vi "A1_图像处理结果.vi"(0 "Image In":T3(plugin-control), 5 "ParamsUI":T1={"IsNorImage"=FALSE, "Exposure Values"=0, "ImagePath"=path "", " Step1 Range"={"Lower value"=117.0, "Upper value"=255.0}, "Step2 Selection Values"=[{"Measurement Parameter"=5, "Range Lower Value"=223.0, "Range Upper Value"=707.0, "Range"=FALSE, "Measurement Type"=FALSE}, {"Measurement Parameter"=4, "Range Lower Value"=0.0, "Range Upper Value"=0.0, "Range"=FALSE, "Measurement Type"=FALSE}], "Step2 Keep/Remove Particles"=TRUE, "Step3 Selection Values 2"=[{"Measurement Parameter"=35, "Range Lower Value"=700.0, "Range Upper Value"=16882.0, "Range"=FALSE, "Measurement Type"=FALSE}], "Step3Keep/Remove Particles 2"=TRUE, "Step4 Selection Values"=[{"Measurement Parameter"=35, "Range Lower Value"=0.0, "Range Upper Value"=393.0, "Range"=FALSE, "Measurement Type"=FALSE}], "Step4 Keep/Remove Particles"=TRUE, "Step5Selection Values"=[{"Measurement Parameter"=2, "Range Lower Value"=564.0, "Range Upper Value"=2005.0, "Range"=FALSE, "Measurement Type"=FALSE}], "Step5 Keep/Remove Particles"=TRUE, "Inspection Number"=0} caption="参数界面" {"Step5Selection Values"."Measurement Parameter" items=["Center of Mass X", "Center of Mass Y", "First Pixel X", "First Pixel Y", "Bounding Rect Left", "Bounding Rect Top", "Bounding Rect Right", "Bounding Rect Bottom", "Max Feret Diameter Start X", "Max Feret Diameter Start Y", "Max Feret Diameter End X", "Max Feret Diameter End Y", "Max Horiz. Segment Length Left", "Max Horiz. Segment Length Right", "Max Horiz. Segment Length Row", "-", "Bounding Rect Width", "Bounding Rect Height", "Bounding Rect Diagonal", "Perimeter", "Convex Hull Perimeter", "Holes' Perimeter", "Max Feret Diameter", "Equivalent Ellipse Major Axis", "Equivalent Ellipse Minor Axis", "Equivalent Ellipse Minor Axis (Feret)", "Equivalent Rect Long Side", "Equivalent Rect Short Side", "Equivalent Rect Diagonal", "Equivalent Rect Short Side (Feret)", "Average Horiz. Segment Length", "Average Vert. Segment Length", "Hydraulic Radius", "Waddel Disk Diameter", "-", "Area", "Holes' Area", "Particle & Holes' Area", "Convex Hull Area", "Image Area", "-", "Number of Holes", "Number of Horiz. Segments", "Number of Vert. Segments", "-", "Orientation", "Max Feret Diameter Orientation", "-", "% Area/Image Area", "% Area/(Particle & Holes' Area)", "Ratio of Equivalent Ellipse Axes", "Ratio of Equivalent Rect Sides", "-", "Elongation Factor", "Compactness Factor", "Heywood Circularity Factor", "Type Factor", "-", "Sum X", "Sum Y", "Sum XX", "Sum XY", "Sum YY", "Sum XXX", "Sum XXY", "Sum XYY", "Sum YYY", "-", "Moment of Inertia XX", "Moment of Inertia XY", "Moment of Inertia YY", "Moment of Inertia XXX", "Moment of Inertia XXY", "Moment of Inertia XYY", "Moment of Inertia YYY", "Norm. Moment of Inertia XX", "Norm. Moment of Inertia XY", "Norm. Moment of Inertia YY", "Norm. Moment of Inertia XXX", "Norm. Moment of Inertia XXY", "Norm. Moment of Inertia XYY", "Norm. Moment of Inertia YYY", "Hu Moment 1", "Hu Moment 2", "Hu Moment 3", "Hu Moment 4", "Hu Moment 5", "Hu Moment 6", "Hu Moment 7"]; "Step4 Selection Values"."Measurement Parameter" items=["Center of Mass X", "Center of Mass Y", "First Pixel X", "First Pixel Y", "Bounding Rect Left", "Bounding Rect Top", "Bounding Rect Right", "Bounding Rect Bottom", "Max Feret Diameter Start X", "Max Feret Diameter Start Y", "Max Feret Diameter End X", "Max Feret Diameter End Y", "Max Horiz. Segment Length Left", "Max Horiz. Segment Length Right", "Max Horiz. Segment Length Row", "-", "Bounding Rect Width", "Bounding Rect Height", "Bounding Rect Diagonal", "Perimeter", "Convex Hull Perimeter", "Holes' Perimeter", "Max Feret Diameter", "Equivalent Ellipse Major Axis", "Equivalent Ellipse Minor Axis", "Equivalent Ellipse Minor Axis (Feret)", "Equivalent Rect Long Side", "Equivalent Rect Short Side", "Equivalent Rect Diagonal", "Equivalent Rect Short Side (Feret)", "Average Horiz. Segment Length", "Average Vert. Segment Length", "Hydraulic Radius", "Waddel Disk Diameter", "-", "Area", "Holes' Area", "Particle & Holes' Area", "Convex Hull Area", "Image Area", "-", "Number of Holes", "Number of Horiz. Segments", "Number of Vert. Segments", "-", "Orientation", "Max Feret Diameter Orientation", "-", "% Area/Image Area", "% Area/(Particle & Holes' Area)", "Ratio of Equivalent Ellipse Axes", "Ratio of Equivalent Rect Sides", "-", "Elongation Factor", "Compactness Factor", "Heywood Circularity Factor", "Type Factor", "-", "Sum X", "Sum Y", "Sum XX", "Sum XY", "Sum YY", "Sum XXX", "Sum XXY", "Sum XYY", "Sum YYY", "-", "Moment of Inertia XX", "Moment of Inertia XY", "Moment of Inertia YY", "Moment of Inertia XXX", "Moment of Inertia XXY", "Moment of Inertia XYY", "Moment of Inertia YYY", "Norm. Moment of Inertia XX", "Norm. Moment of Inertia XY", "Norm. Moment of Inertia YY", "Norm. Moment of Inertia XXX", "Norm. Moment of Inertia XXY", "Norm. Moment of Inertia XYY", "Norm. Moment of Inertia YYY", "Hu Moment 1", "Hu Moment 2", "Hu Moment 3", "Hu Moment 4", "Hu Moment 5", "Hu Moment 6", "Hu Moment 7"]; "Step3 Selection Values 2"."Measurement Parameter" items=["Center of Mass X", "Center of Mass Y", "First Pixel X", "First Pixel Y", "Bounding Rect Left", "Bounding Rect Top", "Bounding Rect Right", "Bounding Rect Bottom", "Max Feret Diameter Start X", "Max Feret Diameter Start Y", "Max Feret Diameter End X", "Max Feret Diameter End Y", "Max Horiz. Segment Length Left", "Max Horiz. Segment Length Right", "Max Horiz. Segment Length Row", "-", "Bounding Rect Width", "Bounding Rect Height", "Bounding Rect Diagonal", "Perimeter", "Convex Hull Perimeter", "Holes' Perimeter", "Max Feret Diameter", "Equivalent Ellipse Major Axis", "Equivalent Ellipse Minor Axis", "Equivalent Ellipse Minor Axis (Feret)", "Equivalent Rect Long Side", "Equivalent Rect Short Side", "Equivalent Rect Diagonal", "Equivalent Rect Short Side (Feret)", "Average Horiz. Segment Length", "Average Vert. Segment Length", "Hydraulic Radius", "Waddel Disk Diameter", "-", "Area", "Holes' Area", "Particle & Holes' Area", "Convex Hull Area", "Image Area", "-", "Number of Holes", "Number of Horiz. Segments", "Number of Vert. Segments", "-", "Orientation", "Max Feret Diameter Orientation", "-", "% Area/Image Area", "% Area/(Particle & Holes' Area)", "Ratio of Equivalent Ellipse Axes", "Ratio of Equivalent Rect Sides", "-", "Elongation Factor", "Compactness Factor", "Heywood Circularity Factor", "Type Factor", "-", "Sum X", "Sum Y", "Sum XX", "Sum XY", "Sum YY", "Sum XXX", "Sum XXY", "Sum XYY", "Sum YYY", "-", "Moment of Inertia XX", "Moment of Inertia XY", "Moment of Inertia YY", "Moment of Inertia XXX", "Moment of Inertia XXY", "Moment of Inertia XYY", "Moment of Inertia YYY", "Norm. Moment of Inertia XX", "Norm. Moment of Inertia XY", "Norm. Moment of Inertia YY", "Norm. Moment of Inertia XXX", "Norm. Moment of Inertia XXY", "Norm. Moment of Inertia XYY", "Norm. Moment of Inertia YYY", "Hu Moment 1", "Hu Moment 2", "Hu Moment 3", "Hu Moment 4", "Hu Moment 5", "Hu Moment 6", "Hu Moment 7"]; "Step2 Selection Values"."Measurement Parameter" items=["Center of Mass X", "Center of Mass Y", "First Pixel X", "First Pixel Y", "Bounding Rect Left", "Bounding Rect Top", "Bounding Rect Right", "Bounding Rect Bottom", "Max Feret Diameter Start X", "Max Feret Diameter Start Y", "Max Feret Diameter End X", "Max Feret Diameter End Y", "Max Horiz. Segment Length Left", "Max Horiz. Segment Length Right", "Max Horiz. Segment Length Row", "-", "Bounding Rect Width", "Bounding Rect Height", "Bounding Rect Diagonal", "Perimeter", "Convex Hull Perimeter", "Holes' Perimeter", "Max Feret Diameter", "Equivalent Ellipse Major Axis", "Equivalent Ellipse Minor Axis", "Equivalent Ellipse Minor Axis (Feret)", "Equivalent Rect Long Side", "Equivalent Rect Short Side", "Equivalent Rect Diagonal", "Equivalent Rect Short Side (Feret)", "Average Horiz. Segment Length", "Average Vert. Segment Length", "Hydraulic Radius", "Waddel Disk Diameter", "-", "Area", "Holes' Area", "Particle & Holes' Area", "Convex Hull Area", "Image Area", "-", "Number of Holes", "Number of Horiz. Segments", "Number of Vert. Segments", "-", "Orientation", "Max Feret Diameter Orientation", "-", "% Area/Image Area", "% Area/(Particle & Holes' Area)", "Ratio of Equivalent Ellipse Axes", "Ratio of Equivalent Rect Sides", "-", "Elongation Factor", "Compactness Factor", "Heywood Circularity Factor", "Type Factor", "-", "Sum X", "Sum Y", "Sum XX", "Sum XY", "Sum YY", "Sum XXX", "Sum XXY", "Sum XYY", "Sum YYY", "-", "Moment of Inertia XX", "Moment of Inertia XY", "Moment of Inertia YY", "Moment of Inertia XXX", "Moment of Inertia XXY", "Moment of Inertia XYY", "Moment of Inertia YYY", "Norm. Moment of Inertia XX", "Norm. Moment of Inertia XY", "Norm. Moment of Inertia YY", "Norm. Moment of Inertia XXX", "Norm. Moment of Inertia XXY", "Norm. Moment of Inertia XYY", "Norm. Moment of Inertia YYY", "Hu Moment 1", "Hu Moment 2", "Hu Moment 3", "Hu Moment 4", "Hu Moment 5", "Hu Moment 6", "Hu Moment 7"]; "Exposure Values" scale=0.0..200000.0}, 11 "error in":errorcluster) -> (4 "Image Out":T3(plugin-control), 6 "Particle Measurements (Real-World)":dbl[][](array[numeric]) format="%.2f", 15 "error out":errorcluster)   [LabVIEW 2015]
uses:
  <vilib>/vision/NI_Vision_Development_Module.lvlib
panel:
  in  "Step5 Keep/Remove Particles":bool=TRUE
  in  "Step5Selection Values":T2(array[cluster])=[{"Measurement Parameter"=2, "Range Lower Value"=564.0, "Range Upper Value"=2005.0, "Range"=FALSE, "Measurement Type"=FALSE}] {"Measurement Parameter" items=["Center of Mass X", "Center of Mass Y", "First Pixel X", "First Pixel Y", "Bounding Rect Left", "Bounding Rect Top", "Bounding Rect Right", "Bounding Rect Bottom", "Max Feret Diameter Start X", "Max Feret Diameter Start Y", "Max Feret Diameter End X", "Max Feret Diameter End Y", "Max Horiz. Segment Length Left", "Max Horiz. Segment Length Right", "Max Horiz. Segment Length Row", "-", "Bounding Rect Width", "Bounding Rect Height", "Bounding Rect Diagonal", "Perimeter", "Convex Hull Perimeter", "Holes' Perimeter", "Max Feret Diameter", "Equivalent Ellipse Major Axis", "Equivalent Ellipse Minor Axis", "Equivalent Ellipse Minor Axis (Feret)", "Equivalent Rect Long Side", "Equivalent Rect Short Side", "Equivalent Rect Diagonal", "Equivalent Rect Short Side (Feret)", "Average Horiz. Segment Length", "Average Vert. Segment Length", "Hydraulic Radius", "Waddel Disk Diameter", "-", "Area", "Holes' Area", "Particle & Holes' Area", "Convex Hull Area", "Image Area", "-", "Number of Holes", "Number of Horiz. Segments", "Number of Vert. Segments", "-", "Orientation", "Max Feret Diameter Orientation", "-", "% Area/Image Area", "% Area/(Particle & Holes' Area)", "Ratio of Equivalent Ellipse Axes", "Ratio of Equivalent Rect Sides", "-", "Elongation Factor", "Compactness Factor", "Heywood Circularity Factor", "Type Factor", "-", "Sum X", "Sum Y", "Sum XX", "Sum XY", "Sum YY", "Sum XXX", "Sum XXY", "Sum XYY", "Sum YYY", "-", "Moment of Inertia XX", "Moment of Inertia XY", "Moment of Inertia YY", "Moment of Inertia XXX", "Moment of Inertia XXY", "Moment of Inertia XYY", "Moment of Inertia YYY", "Norm. Moment of Inertia XX", "Norm. Moment of Inertia XY", "Norm. Moment of Inertia YY", "Norm. Moment of Inertia XXX", "Norm. Moment of Inertia XXY", "Norm. Moment of Inertia XYY", "Norm. Moment of Inertia YYY", "Hu Moment 1", "Hu Moment 2", "Hu Moment 3", "Hu Moment 4", "Hu Moment 5", "Hu Moment 6", "Hu Moment 7"]}
  in  "Step4Keep/Remove Particles":bool=TRUE
  in  "Step4 Selection Values":T2(array[cluster])=[{"Measurement Parameter"=35, "Range Lower Value"=0.0, "Range Upper Value"=393.0, "Range"=FALSE, "Measurement Type"=FALSE}] {"Measurement Parameter" items=["Center of Mass X", "Center of Mass Y", "First Pixel X", "First Pixel Y", "Bounding Rect Left", "Bounding Rect Top", "Bounding Rect Right", "Bounding Rect Bottom", "Max Feret Diameter Start X", "Max Feret Diameter Start Y", "Max Feret Diameter End X", "Max Feret Diameter End Y", "Max Horiz. Segment Length Left", "Max Horiz. Segment Length Right", "Max Horiz. Segment Length Row", "-", "Bounding Rect Width", "Bounding Rect Height", "Bounding Rect Diagonal", "Perimeter", "Convex Hull Perimeter", "Holes' Perimeter", "Max Feret Diameter", "Equivalent Ellipse Major Axis", "Equivalent Ellipse Minor Axis", "Equivalent Ellipse Minor Axis (Feret)", "Equivalent Rect Long Side", "Equivalent Rect Short Side", "Equivalent Rect Diagonal", "Equivalent Rect Short Side (Feret)", "Average Horiz. Segment Length", "Average Vert. Segment Length", "Hydraulic Radius", "Waddel Disk Diameter", "-", "Area", "Holes' Area", "Particle & Holes' Area", "Convex Hull Area", "Image Area", "-", "Number of Holes", "Number of Horiz. Segments", "Number of Vert. Segments", "-", "Orientation", "Max Feret Diameter Orientation", "-", "% Area/Image Area", "% Area/(Particle & Holes' Area)", "Ratio of Equivalent Ellipse Axes", "Ratio of Equivalent Rect Sides", "-", "Elongation Factor", "Compactness Factor", "Heywood Circularity Factor", "Type Factor", "-", "Sum X", "Sum Y", "Sum XX", "Sum XY", "Sum YY", "Sum XXX", "Sum XXY", "Sum XYY", "Sum YYY", "-", "Moment of Inertia XX", "Moment of Inertia XY", "Moment of Inertia YY", "Moment of Inertia XXX", "Moment of Inertia XXY", "Moment of Inertia XYY", "Moment of Inertia YYY", "Norm. Moment of Inertia XX", "Norm. Moment of Inertia XY", "Norm. Moment of Inertia YY", "Norm. Moment of Inertia XXX", "Norm. Moment of Inertia XXY", "Norm. Moment of Inertia XYY", "Norm. Moment of Inertia YYY", "Hu Moment 1", "Hu Moment 2", "Hu Moment 3", "Hu Moment 4", "Hu Moment 5", "Hu Moment 6", "Hu Moment 7"]}
  in  "Step3Keep/Remove Particles 2":bool=TRUE
  in  "Step3 Selection Values 2":T2(array[cluster])=[{"Measurement Parameter"=35, "Range Lower Value"=700.0, "Range Upper Value"=16882.0, "Range"=FALSE, "Measurement Type"=FALSE}] {"Measurement Parameter" items=["Center of Mass X", "Center of Mass Y", "First Pixel X", "First Pixel Y", "Bounding Rect Left", "Bounding Rect Top", "Bounding Rect Right", "Bounding Rect Bottom", "Max Feret Diameter Start X", "Max Feret Diameter Start Y", "Max Feret Diameter End X", "Max Feret Diameter End Y", "Max Horiz. Segment Length Left", "Max Horiz. Segment Length Right", "Max Horiz. Segment Length Row", "-", "Bounding Rect Width", "Bounding Rect Height", "Bounding Rect Diagonal", "Perimeter", "Convex Hull Perimeter", "Holes' Perimeter", "Max Feret Diameter", "Equivalent Ellipse Major Axis", "Equivalent Ellipse Minor Axis", "Equivalent Ellipse Minor Axis (Feret)", "Equivalent Rect Long Side", "Equivalent Rect Short Side", "Equivalent Rect Diagonal", "Equivalent Rect Short Side (Feret)", "Average Horiz. Segment Length", "Average Vert. Segment Length", "Hydraulic Radius", "Waddel Disk Diameter", "-", "Area", "Holes' Area", "Particle & Holes' Area", "Convex Hull Area", "Image Area", "-", "Number of Holes", "Number of Horiz. Segments", "Number of Vert. Segments", "-", "Orientation", "Max Feret Diameter Orientation", "-", "% Area/Image Area", "% Area/(Particle & Holes' Area)", "Ratio of Equivalent Ellipse Axes", "Ratio of Equivalent Rect Sides", "-", "Elongation Factor", "Compactness Factor", "Heywood Circularity Factor", "Type Factor", "-", "Sum X", "Sum Y", "Sum XX", "Sum XY", "Sum YY", "Sum XXX", "Sum XXY", "Sum XYY", "Sum YYY", "-", "Moment of Inertia XX", "Moment of Inertia XY", "Moment of Inertia YY", "Moment of Inertia XXX", "Moment of Inertia XXY", "Moment of Inertia XYY", "Moment of Inertia YYY", "Norm. Moment of Inertia XX", "Norm. Moment of Inertia XY", "Norm. Moment of Inertia YY", "Norm. Moment of Inertia XXX", "Norm. Moment of Inertia XXY", "Norm. Moment of Inertia XYY", "Norm. Moment of Inertia YYY", "Hu Moment 1", "Hu Moment 2", "Hu Moment 3", "Hu Moment 4", "Hu Moment 5", "Hu Moment 6", "Hu Moment 7"]}
  in  "Step2 Keep/Remove Particles":bool=TRUE
  in  "Step2 Selection Values":T2(array[cluster])=[{"Measurement Parameter"=5, "Range Lower Value"=223.0, "Range Upper Value"=707.0, "Range"=FALSE, "Measurement Type"=FALSE}, {"Measurement Parameter"=4, "Range Lower Value"=0.0, "Range Upper Value"=0.0, "Range"=FALSE, "Measurement Type"=FALSE}] {"Measurement Parameter" items=["Center of Mass X", "Center of Mass Y", "First Pixel X", "First Pixel Y", "Bounding Rect Left", "Bounding Rect Top", "Bounding Rect Right", "Bounding Rect Bottom", "Max Feret Diameter Start X", "Max Feret Diameter Start Y", "Max Feret Diameter End X", "Max Feret Diameter End Y", "Max Horiz. Segment Length Left", "Max Horiz. Segment Length Right", "Max Horiz. Segment Length Row", "-", "Bounding Rect Width", "Bounding Rect Height", "Bounding Rect Diagonal", "Perimeter", "Convex Hull Perimeter", "Holes' Perimeter", "Max Feret Diameter", "Equivalent Ellipse Major Axis", "Equivalent Ellipse Minor Axis", "Equivalent Ellipse Minor Axis (Feret)", "Equivalent Rect Long Side", "Equivalent Rect Short Side", "Equivalent Rect Diagonal", "Equivalent Rect Short Side (Feret)", "Average Horiz. Segment Length", "Average Vert. Segment Length", "Hydraulic Radius", "Waddel Disk Diameter", "-", "Area", "Holes' Area", "Particle & Holes' Area", "Convex Hull Area", "Image Area", "-", "Number of Holes", "Number of Horiz. Segments", "Number of Vert. Segments", "-", "Orientation", "Max Feret Diameter Orientation", "-", "% Area/Image Area", "% Area/(Particle & Holes' Area)", "Ratio of Equivalent Ellipse Axes", "Ratio of Equivalent Rect Sides", "-", "Elongation Factor", "Compactness Factor", "Heywood Circularity Factor", "Type Factor", "-", "Sum X", "Sum Y", "Sum XX", "Sum XY", "Sum YY", "Sum XXX", "Sum XXY", "Sum XYY", "Sum YYY", "-", "Moment of Inertia XX", "Moment of Inertia XY", "Moment of Inertia YY", "Moment of Inertia XXX", "Moment of Inertia XXY", "Moment of Inertia XYY", "Moment of Inertia YYY", "Norm. Moment of Inertia XX", "Norm. Moment of Inertia XY", "Norm. Moment of Inertia YY", "Norm. Moment of Inertia XXX", "Norm. Moment of Inertia XXY", "Norm. Moment of Inertia XYY", "Norm. Moment of Inertia YYY", "Hu Moment 1", "Hu Moment 2", "Hu Moment 3", "Hu Moment 4", "Hu Moment 5", "Hu Moment 6", "Hu Moment 7"]}
  in  "Step1 Range In":cluster{"Lower value":sgl, "Upper value":sgl}={"Lower value"=117.0, "Upper value"=255.0}
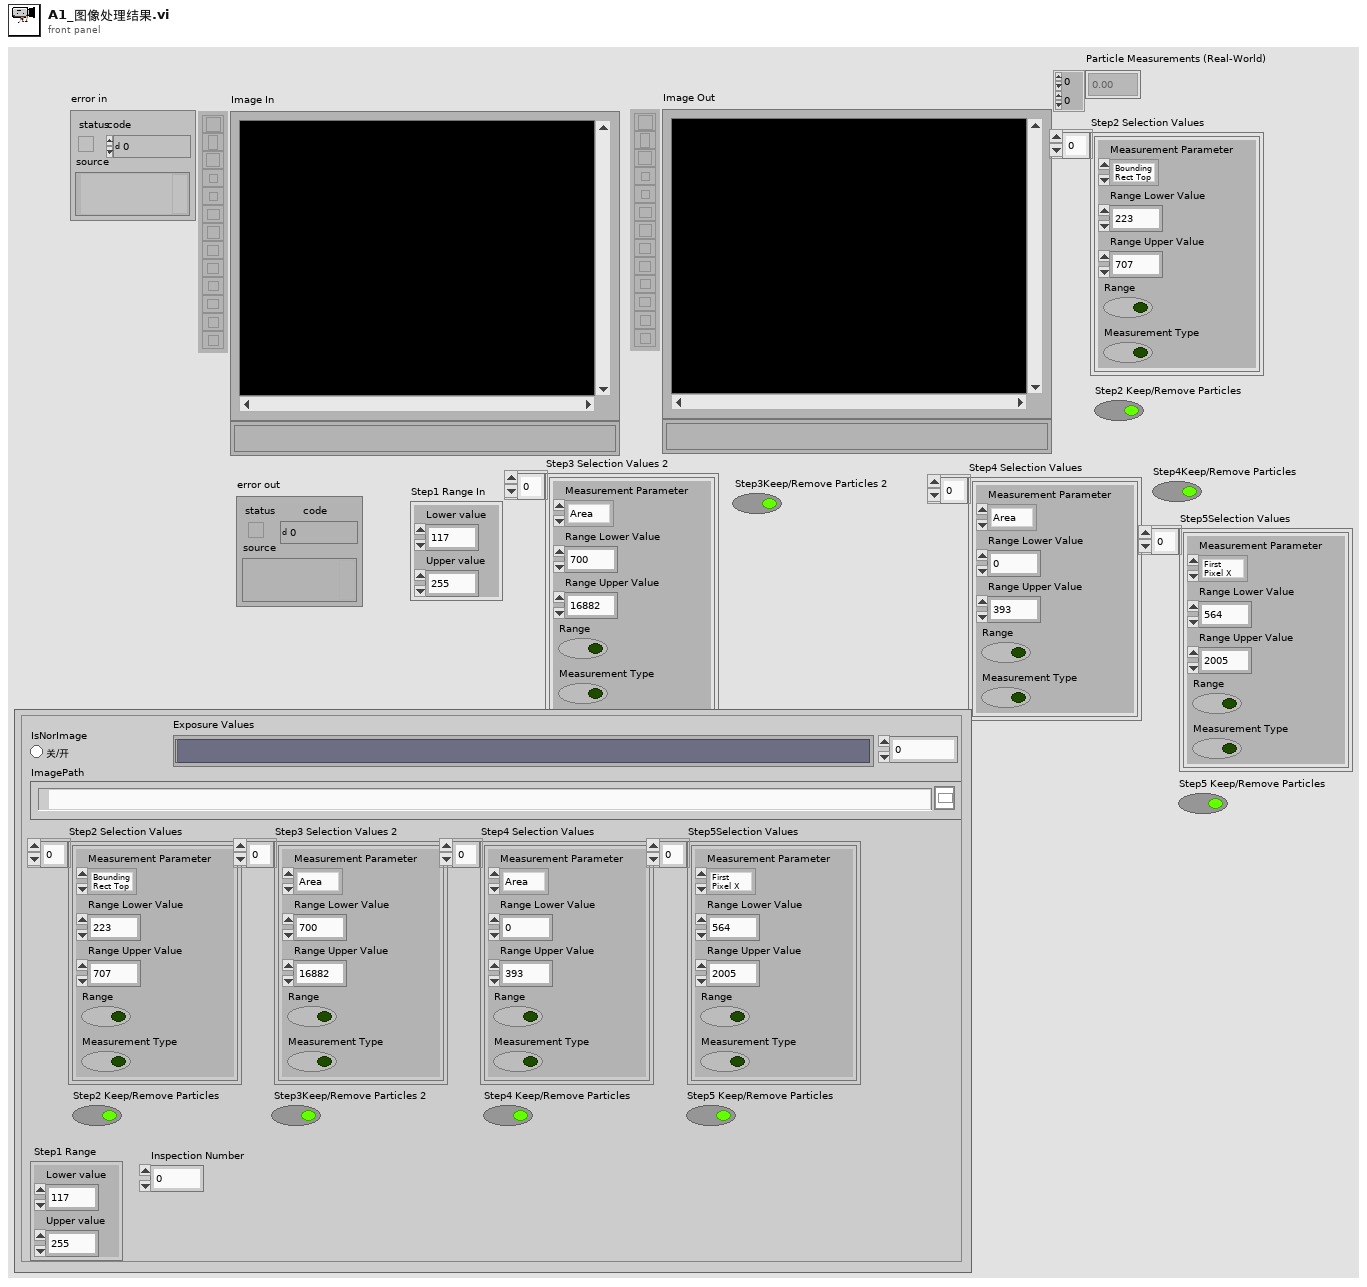
[diagram p1: front panel]
types:
  T1 = cluster{"IsNorImage":bool, "Exposure Values":u32, "ImagePath":path, " Step1 Range":cluster{"Lower value":sgl, "Upper value":sgl}, "Step2 Selection Values":cluster{"Measurement Parameter":i32, "Range Lower Value":dbl, "Range Upper Value":dbl, "Range":bool, "Measurement Type":bool}[], "Step2 Keep/Remove Particles":bool, "Step3 Selection Values 2":cluster{"Measurement Parameter":i32, "Range Lower Value":dbl, "Range Upper Value":dbl, "Range":bool, "Measurement Type":bool}[], "Step3Keep/Remove Particles 2":bool, "Step4 Selection Values":cluster{"Measurement Parameter":i32, "Range Lower Value":dbl, "Range Upper Value":dbl, "Range":bool, "Measurement Type":bool}[], "Step4 Keep/Remove Particles":bool, "Step5Selection Values":cluster{"Measurement Parameter":i32, "Range Lower Value":dbl, "Range Upper Value":dbl, "Range":bool, "Measurement Type":bool}[], "Step5 Keep/Remove Particles":bool, "Inspection Number":i32}
  T2 = cluster{"Measurement Parameter":i32, "Range Lower Value":dbl, "Range Upper Value":dbl, "Range":bool, "Measurement Type":bool}[]
  T3 = typedef "IMAQ Image.ctl" = refnum<image>
  T4 = enum32{"Differentiation", "Gradient", "Prewitt", "Roberts", "Sigma", "Sobel"}
  T5 = enum32{"AutoM", "Close", "Dilate", "Erode", "Gradient", "Gradient in", "Gradient out", "HitMiss", "Open", "PClose", "POpen", "Thick", "Thin"}
  T6 = cluster{"histogram":u32[], "Minimal Value":sgl, "Maximal Value":sgl, "Starting Value":sgl, "Interval Width":sgl, "Mean Value":sgl, "Standard  Variation":sgl, "Area (pixels)":i32}
  T7 = typedef "Image Type" = u32
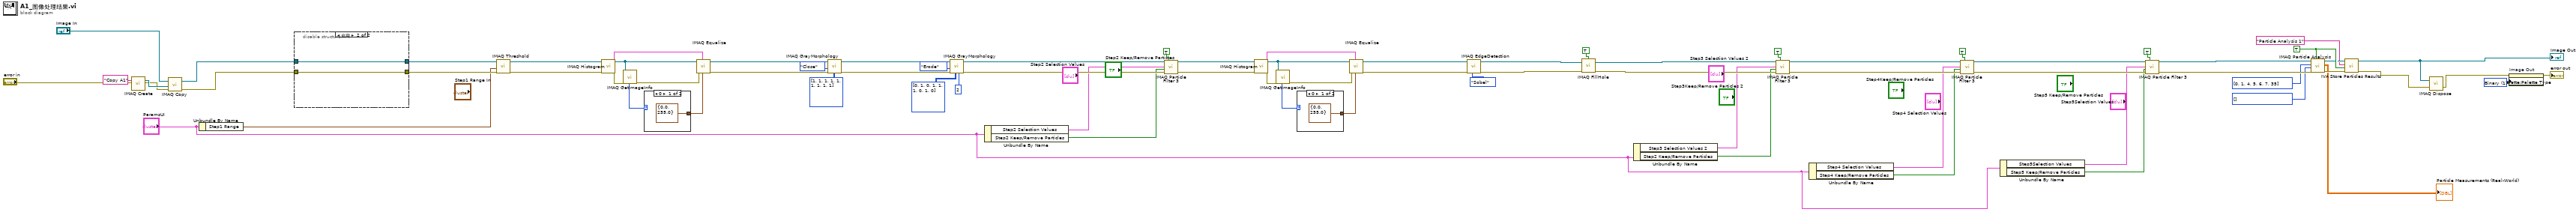
[diagram p0: block diagram]
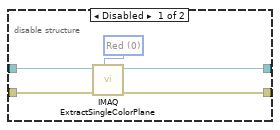
[diagram p2: hidden frame]
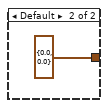
[diagram p3: hidden frame]
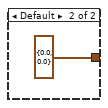
[diagram p4: hidden frame]
diagram:
  w21 = u32 1 items=["Grayscale", "Binary", "Gradient", "Rainbow", "Temperature", "User Defined", "Binary 16 Bit", "Gradient 16 Bit", "Rainbow 16 Bit", "Temperature 16 Bit", "User Defined 16 Bit"] ("Palette Type")
  w28 = i32[] [] items=["Center of Mass X", "Center of Mass Y", "First Pixel X", "First Pixel Y", "Bounding Rect Left", "Bounding Rect Top", "Bounding Rect Right", "Bounding Rect Bottom", "Max Feret Diameter Start X", "Max Feret Diameter Start Y", "Max Feret Diameter End X", "Max Feret Diameter End Y", "Max Horiz. Segment Length Left", "Max Horiz. Segment Length Right", "Max Horiz. Segment Length Row", "-", "Bounding Rect Width", "Bounding Rect Height", "Bounding Rect Diagonal", "Perimeter", "Convex Hull Perimeter", "Holes' Perimeter", "Max Feret Diameter", "Equivalent Ellipse Major Axis", "Equivalent Ellipse Minor Axis", "Equivalent Ellipse Minor Axis (Feret)", "Equivalent Rect Long Side", "Equivalent Rect Short Side", "Equivalent Rect Diagonal", "Equivalent Rect Short Side (Feret)", "Average Horiz. Segment Length", "Average Vert. Segment Length", "Hydraulic Radius", "Waddel Disk Diameter", "-", "Area", "Holes' Area", "Particle & Holes' Area", "Convex Hull Area", "Image Area", "-", "Number of Holes", "Number of Horiz. Segments", "Number of Vert. Segments", "-", "Orientation", "Max Feret Diameter Orientation", "-", "% Area/Image Area", "% Area/(Particle & Holes' Area)", "Ratio of Equivalent Ellipse Axes", "Ratio of Equivalent Rect Sides", "-", "Elongation Factor", "Compactness Factor", "Heywood Circularity Factor", "Type Factor", "-", "Sum X", "Sum Y", "Sum XX", "Sum XY", "Sum YY", "Sum XXX", "Sum XXY", "Sum XYY", "Sum YYY", "-", "Moment of Inertia XX", "Moment of Inertia XY", "Moment of Inertia YY", "Moment of Inertia XXX", "Moment of Inertia XXY", "Moment of Inertia XYY", "Moment of Inertia YYY", "Norm. Moment of Inertia XX", "Norm. Moment of Inertia XY", "Norm. Moment of Inertia YY", "Norm. Moment of Inertia XXX", "Norm. Moment of Inertia XXY", "Norm. Moment of Inertia XYY", "Norm. Moment of Inertia YYY", "Hu Moment 1", "Hu Moment 2", "Hu Moment 3", "Hu Moment 4", "Hu Moment 5", "Hu Moment 6", "Hu Moment 7"] ("Real-World Measurements")
  w29 = i32[] [0, 1, 4, 5, 6, 7, 35] items=["Center of Mass X", "Center of Mass Y", "First Pixel X", "First Pixel Y", "Bounding Rect Left", "Bounding Rect Top", "Bounding Rect Right", "Bounding Rect Bottom", "Max Feret Diameter Start X", "Max Feret Diameter Start Y", "Max Feret Diameter End X", "Max Feret Diameter End Y", "Max Horiz. Segment Length Left", "Max Horiz. Segment Length Right", "Max Horiz. Segment Length Row", "-", "Bounding Rect Width", "Bounding Rect Height", "Bounding Rect Diagonal", "Perimeter", "Convex Hull Perimeter", "Holes' Perimeter", "Max Feret Diameter", "Equivalent Ellipse Major Axis", "Equivalent Ellipse Minor Axis", "Equivalent Ellipse Minor Axis (Feret)", "Equivalent Rect Long Side", "Equivalent Rect Short Side", "Equivalent Rect Diagonal", "Equivalent Rect Short Side (Feret)", "Average Horiz. Segment Length", "Average Vert. Segment Length", "Hydraulic Radius", "Waddel Disk Diameter", "-", "Area", "Holes' Area", "Particle & Holes' Area", "Convex Hull Area", "Image Area", "-", "Number of Holes", "Number of Horiz. Segments", "Number of Vert. Segments", "-", "Orientation", "Max Feret Diameter Orientation", "-", "% Area/Image Area", "% Area/(Particle & Holes' Area)", "Ratio of Equivalent Ellipse Axes", "Ratio of Equivalent Rect Sides", "-", "Elongation Factor", "Compactness Factor", "Heywood Circularity Factor", "Type Factor", "-", "Sum X", "Sum Y", "Sum XX", "Sum XY", "Sum YY", "Sum XXX", "Sum XXY", "Sum XYY", "Sum YYY", "-", "Moment of Inertia XX", "Moment of Inertia XY", "Moment of Inertia YY", "Moment of Inertia XXX", "Moment of Inertia XXY", "Moment of Inertia XYY", "Moment of Inertia YYY", "Norm. Moment of Inertia XX", "Norm. Moment of Inertia XY", "Norm. Moment of Inertia YY", "Norm. Moment of Inertia XXX", "Norm. Moment of Inertia XXY", "Norm. Moment of Inertia XYY", "Norm. Moment of Inertia YYY", "Hu Moment 1", "Hu Moment 2", "Hu Moment 3", "Hu Moment 4", "Hu Moment 5", "Hu Moment 6", "Hu Moment 7"] ("Pixel Measurements")
  w26 = TRUE ("Connectivity 4/8 (8)")
  n1 = call "IMAQ Create"("Image Name"="Copy A1") -> ("New Image"=w19:T3)  [unwired: 4 in, 1 out]
  n2 = call "IMAQ Copy"("error in (no error)"="error in", "Image Dst"=w19, "Image Src"="Image In") -> ("error out"=w16:errorcluster, "Image Dst Out"=w17:T3)  [unwired: 3 in]
  n3 = Unbundle By Name("ParamsUI") -> ("Step1 Range"=w10:cluster{"Lower value":sgl, "Upper value":sgl})
  n4 = disable-structure shown="启用" {
    disable-tunnel: [w77 w79] -> w73
    disable-tunnel: [w76 w80] -> w72
    disable-tunnel: w17 -> [w75 w80]
    disable-tunnel: w16 -> [w74 w79]
    frame Disabled {
      w78 = 0 items=["Red", "Green", "Blue", "Hue", "Saturation", "Luminance", "Value", "Intensity"] ("Color Plane")
      n5 = call "IMAQ ExtractSingleColorPlane"("Color Plane"=w78, "error in (no error)"=w74, "Image Src"=w75) -> ("error out"=w77:errorcluster, "Image Dst Out"=w76:T3)  [unwired: 1 in, 6 out]
    }
    frame Enabled {
    }
  }
  n6 = call "IMAQ Threshold"("error in (no error)"=w73, "Range"=w10, "Image Src"=w72) -> ("error out"=w71:errorcluster, "Image Dst Out"=w67:T3)  [unwired: 3 in, 4 out]
  n7 = call "IMAQ Histogram"("error in (no error)"=w71, "Image"=w67) -> ("error out"=w66:errorcluster, "Histogram Report"=w69:T6)  [unwired: 3 in, 5 out]
  n8 = call "IMAQ GetImageInfo"("error in (no error)"=w66, "Image"=w67) -> ("error out"=w65:errorcluster, "Image Type"=w68:T7)  [unwired: 8 out]
  n9 = case "条件结构" shown="0" w68 {
    tunnel: [cluster{"Minimum":sgl, "Maximum":sgl} {"Minimum"=0.0, "Maximum"=255.0} ("Range") cluster{"Minimum":sgl, "Maximum":sgl} {"Minimum"=0.0, "Maximum"=0.0} ("Range")] -> w64
    frame 0 {
    }
    frame Default {
    }
  }
  n10 = call "IMAQ Equalize"("Range"=w64, "Histogram Report"=w69, "error in (no error)"=w65, "Image Src"=w67) -> ("error out"=w70:errorcluster, "Image Dst Out"=w61:T3)  [unwired: 2 in, 4 out]
  n11 = call "IMAQ GrayMorphology"("Structuring Element"=i32[][] [[1, 1, 1], [1, 1, 1], [1, 1, 1]], "error in (no error)"=w70, "Operation"=T5."Close", "Image Src"=w61) -> ("error out"=w60:errorcluster, "Image Dst Out"=w57:T3)  [unwired: 3 in, 3 out]
  n12 = call "IMAQ GrayMorphology"("Number of iterations (1)"=2, "Structuring Element"=i32[][] [[0, 1, 0], [1, 1, 1], [0, 1, 0]], "error in (no error)"=w60, "Operation"=T5."Erode", "Image Src"=w57) -> ("error out"=w56:errorcluster, "Image Dst Out"=w52:T3)  [unwired: 2 in, 3 out]
  n13 = Unbundle By Name("ParamsUI") -> ("Step2 Selection Values"=w9:T2, "Step2 Keep/Remove Particles"=w8:bool)
  n14 = call "IMAQ Particle Filter 3"("Image Src"=w52, "Connectivity 4/8 (8)"=TRUE, "Selection Values"=w9, "Keep/Remove Particles (F)"=w8, "error in (no error)"=w56) -> ("Image Dst Out"=w48:T3, "error out"=w53:errorcluster)  [unwired: 4 in, 5 out]
  n15 = call "IMAQ Histogram"("error in (no error)"=w53, "Image"=w48) -> ("error out"=w47:errorcluster, "Histogram Report"=w50:T6)  [unwired: 3 in, 5 out]
  n16 = call "IMAQ GetImageInfo"("error in (no error)"=w47, "Image"=w48) -> ("error out"=w46:errorcluster, "Image Type"=w49:T7)  [unwired: 8 out]
  n17 = case "条件结构" shown="0" w49 {
    tunnel: [cluster{"Minimum":sgl, "Maximum":sgl} {"Minimum"=0.0, "Maximum"=255.0} ("Range") cluster{"Minimum":sgl, "Maximum":sgl} {"Minimum"=0.0, "Maximum"=0.0} ("Range")] -> w45
    frame 0 {
    }
    frame Default {
    }
  }
  n18 = call "IMAQ Equalize"("Range"=w45, "Histogram Report"=w50, "error in (no error)"=w46, "Image Src"=w48) -> ("error out"=w51:errorcluster, "Image Dst Out"=w43:T3)  [unwired: 2 in, 4 out]
  n19 = call "IMAQ EdgeDetection"("Method"=T4."Sobel", "error in (no error)"=w51, "Image Src"=w43) -> ("error out"=w42:errorcluster, "Image Dst Out"=w40:T3)  [unwired: 3 in, 4 out]
  n20 = call "IMAQ FillHole"("error in (no error)"=w42, "Image Src"=w40, "Connectivity 4/8 (8)"=TRUE) -> ("error out"=w39:errorcluster, "Image Dst Out"=w36:T3)  [unwired: 1 in, 2 out]
  n21 = Unbundle By Name("ParamsUI") -> ("Step3 Selection Values 2"=w7:T2, "Step2 Keep/Remove Particles"=w6:bool)
  n22 = call "IMAQ Particle Filter 3"("Image Src"=w36, "Connectivity 4/8 (8)"=TRUE, "Selection Values"=w7, "Keep/Remove Particles (F)"=w6, "error in (no error)"=w39) -> ("Image Dst Out"=w33:T3, "error out"=w37:errorcluster)  [unwired: 4 in, 5 out]
  n23 = Unbundle By Name("ParamsUI") -> ("Step4 Selection Values"=w5:T2, "Step4 Keep/Remove Particles"=w4:bool)
  n24 = call "IMAQ Particle Filter 3"("Image Src"=w33, "Connectivity 4/8 (8)"=TRUE, "Selection Values"=w5, "Keep/Remove Particles (F)"=w4, "error in (no error)"=w37) -> ("Image Dst Out"=w30:T3, "error out"=w34:errorcluster)  [unwired: 4 in, 5 out]
  n25 = Unbundle By Name("ParamsUI") -> ("Step5Selection Values"=w2:T2, "Step5 Keep/Remove Particles"=w1:bool)
  n26 = call "IMAQ Particle Filter 3"("Image Src"=w30, "Connectivity 4/8 (8)"=TRUE, "Selection Values"=w2, "Keep/Remove Particles (F)"=w1, "error in (no error)"=w34) -> ("Image Dst Out"=w27:T3, "error out"=w31:errorcluster)  [unwired: 4 in, 5 out]
  n27 = call "IMAQ Particle Analysis"("Connectivity 4/8 (8)"=w26, "error in (no error)"=w31, "Real-World Measurements"=w28, "Pixel Measurements"=w29, "Image"=w27) -> ("error out"=w23:errorcluster, "Particle Measurements (Pixels)"=→"Particle Measurements (Real-World)":dbl[][], "Image Out (duplicate)"=w25:T3)  [unwired: 4 out]
  n28 = call <vilib>:"IVA Store Particles Results.vi"("error in (no error)"=w23, "Connectivity 4/8 (8)"=w26, "Step Name"="Particle Analysis 1", "Image in"=w25) -> ("error out"=w13:errorcluster, "Image dup"=w14:T3)  [unwired: 6 out]
  "Image Out" <- w14
  n29 = call "IMAQ Dispose"("Image"=w14, "error in (no error)"=w13) -> ("error out"=w12:errorcluster)  [unwired: 4 in]
  n30 = property on="Image Out" class="ImageControl"(error in=w12, "Palette:Palette Type"=w21) -> (error out=→"error out":errorcluster)  [unwired: 1 in, 1 out]
